vi "getStepNLoopStatus.vi"(0 "Pmx4exSaController in":refnum<class "Pmx4exSaController.lvclass">, 2 "axis":T1, 5 "error in (no error)":errorcluster) -> (14 "Pmx4exSaController out":refnum<class "Pmx4exSaController.lvclass">, 16 "status (out)":T2, 19 "error out":errorcluster)   [LabVIEW 2020, in "classes.lvlib" / "Pmx4exSaController.lvclass"]
doc: "Produced By:\n\n<B>Kod Integrations, LLC</B>\n4835 Marianne Drive\nMount Airy, MD 21771\nhttp://www.kodintegrations.com\nemail: info@kodintegrations.com\nphone: (240) 687-1288"
uses:
  Pmx4exSaController.lvclass
  C:/GEECS/Developers Version/source/Device Drivers/Newmark-NSC-A/Arcus Driver 3.0.0/ArcusUsbComm/classes/Controller/_Controller.lvclass
  step_n_loop_motor_status.ctl
  axis.ctl
  _Controller.lvclass
  common.lvlib
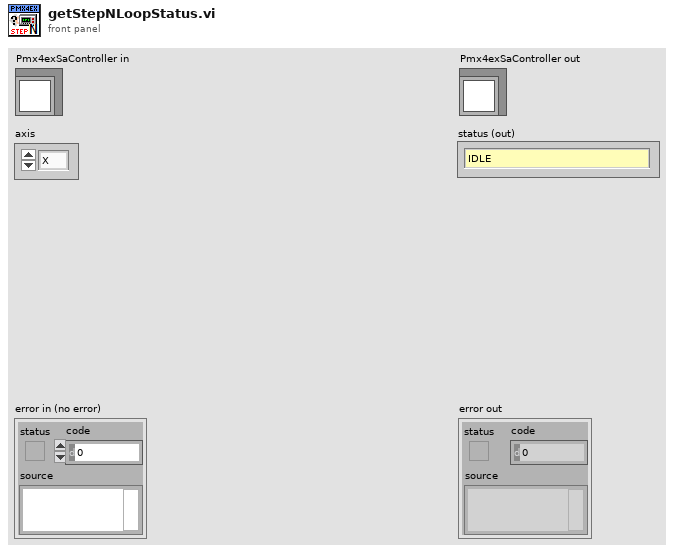
[diagram p1: front panel]
types:
  T1 = typedef "common.lvlib/axis.ctl" = enum16{"X", "Y", "Z", "U"}
  T2 = typedef "common.lvlib/step_n_loop_motor_status.ctl" = enum16{"IDLE", "MOVING", "CORRECTING", "STOPPING", "ABORTING", "JOGGING", "HOMING", "Z-HOMING", "CORRECT_RANGE_ERR", "CORRECT_ATTEMPT_ERR", "STALL_ERR", "LIMIT_ERR", "NA (SNL NOT ENABLED)", "LIMIT_HOMING"}
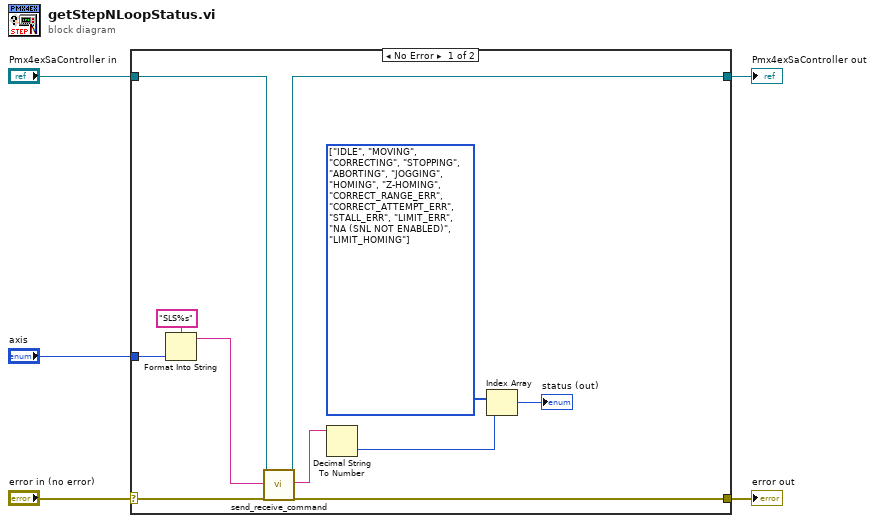
[diagram p0: block diagram]
diagram:
  n1 = case shown="No Error" "error in (no error)" {
    selector: "error in (no error)" -> [w14 w18]
    tunnel: [w13 w18] -> w4
    tunnel: [w10 w17] -> w2
    tunnel: "Pmx4exSaController in" -> [w11 w17]
    tunnel: "axis" -> [w15 _]
    frame No Error {
      w8 = T2[] [enum."IDLE", enum."MOVING", enum."CORRECTING", enum."STOPPING", enum."ABORTING", enum."JOGGING", enum."HOMING", enum."Z-HOMING", enum."CORRECT_RANGE_ERR", enum."CORRECT_ATTEMPT_ERR", enum."STALL_ERR", enum."LIMIT_ERR", enum."NA (SNL NOT ENABLED)", enum."LIMIT_HOMING"] items=["IDLE", "MOVING", "CORRECTING", "STOPPING", "ABORTING", "JOGGING", "HOMING", "Z-HOMING", "CORRECT_RANGE_ERR", "CORRECT_ATTEMPT_ERR", "STALL_ERR", "LIMIT_ERR", "NA (SNL NOT ENABLED)", "LIMIT_HOMING"] ("status (out)")
      n2 = Format Into String(format string="SLS%s", w15) -> (resulting string=w12:string)  [unwired: 2 in, 1 out]
      n3 = call "send_receive_command.vi"("reference (in)"=w11, "ASCII Command (in)"=w12, "error in (no error)"=w14) -> ("reference (out)"=w10:refnum<class "Pmx4exSaController.lvclass">, "response (out)"=w9:string, "error out"=w13:errorcluster)  [unwired: 12 in, 2 out]
      n4 = Decimal String To Number(string=w9) -> (number=w7:i32)  [unwired: 2 in, 1 out]
      n5 = Index Array(array=w8, index=w7) -> (element=→"status (out)":T2)
    }
    frame Error {
    }
  }
  "error out" <- w4
  "Pmx4exSaController out" <- w2
